vi "Read Center (px).vi"(8 "error in (no error)":errorcluster, 11 "Geometric Figure in":refnum<class "UI Object.lvclass">) -> (0 "error out":errorcluster, 2 "Point (px)":T1, 3 "Geometric Figure out":refnum<class "UI Object.lvclass">)   [LabVIEW 2016, in "PacManClasses.lvlib" / "UI Object.lvclass"]
uses:
  UI Object.lvclass
  Generic Controls/Point.ctl
  UI Object.lvclass/UI Object.ctl
  PacManClasses.lvlib
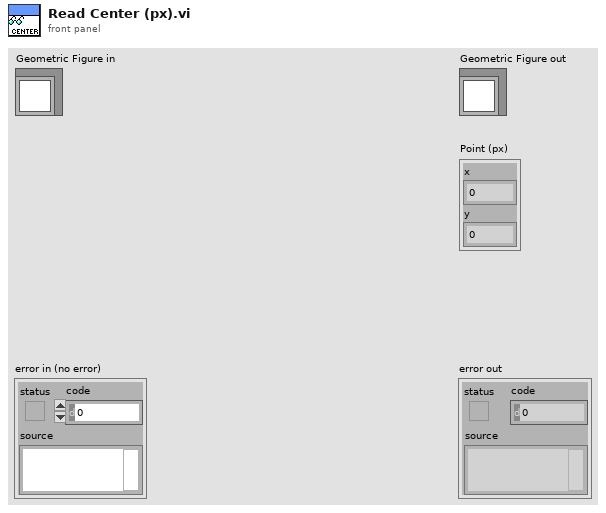
[diagram p1: front panel]
types:
  T1 = typedef "PacManClasses.lvlib/Point.ctl" = cluster{"x":u16, "y":u16}
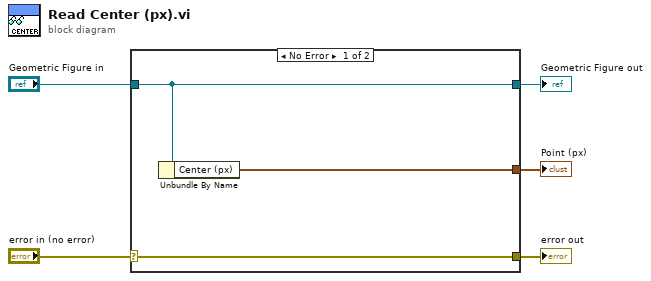
[diagram p0: block diagram]
diagram:
  n1 = case shown="No Error" "error in (no error)" {
    selector: "error in (no error)" -> [w8 w9]
    tunnel: [w8 w9] -> w4
    tunnel: [w7 w10] -> w2
    tunnel: "Geometric Figure in" -> [w7 w10]
    tunnel: [w6 _] -> w1
    frame No Error {
      n2 = Unbundle By Name(w7) -> ("Center (px)"=w6:T1)
    }
    frame Error {
    }
  }
  "error out" <- w4
  "Geometric Figure out" <- w2
  "Point (px)" <- w1
